vi "configureTiming.vi"(8 "error in (no error)":errorcluster, 9 "Routings":cluster{"Master Clock Route":string[]}, 10 "Timing":T1, 11 "DigitalOutput in":refnum<class "DigitalOutput.lvclass">) -> (0 "error out":errorcluster, 3 "DigitalOutput out":refnum<class "DigitalOutput.lvclass">)   [LabVIEW 2011, in "Hardware.lvlib" / "Channels.lvlib" / "DigitalOutput.lvclass"]
uses:
  DigitalOutput.lvclass
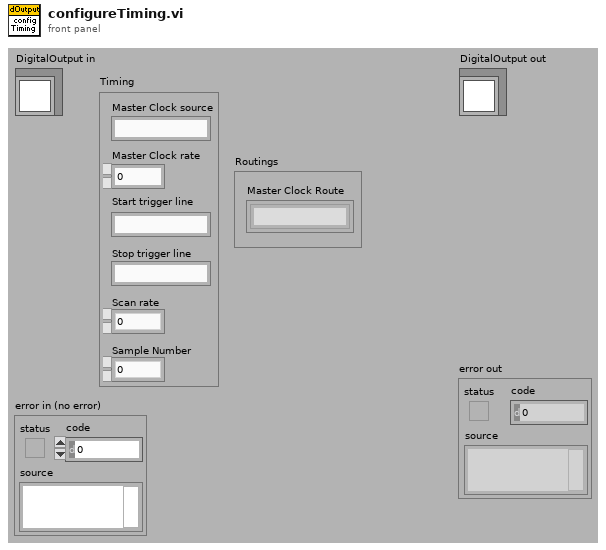
[diagram p1: front panel]
types:
  T1 = cluster{"Master Clock source":string, "Master Clock rate":dbl, "Start trigger line":string, "Scan rate":dbl, "Stop trigger line":string, "Sample Number":dbl}
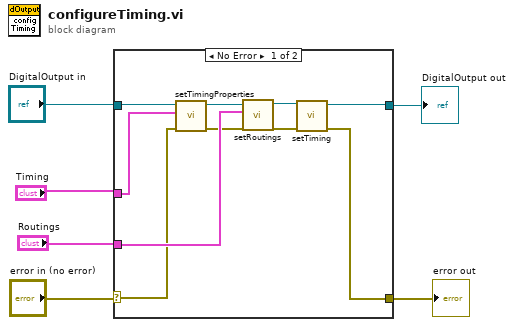
[diagram p0: block diagram]
diagram:
  n1 = case shown="No Error" "error in (no error)" {
    selector: "error in (no error)" -> [w13 w18]
    tunnel: [w7 w18] -> w5
    tunnel: [w8 w17] -> w3
    tunnel: "DigitalOutput in" -> [w12 w17]
    tunnel: "Timing" -> [w11 _]
    tunnel: "Routings" -> [w15 _]
    frame No Error {
      n2 = call-dynamic "setTimingProperties.vi"("error in (no error)"=w13, "Timing"=w11, "DigitalOutput.lvclass in"=w12) -> ("error out"=w14:errorcluster, "DigitalOutput.lvclass out"=w16:refnum<class "DigitalOutput.lvclass">)  [unwired: 7 in]
      n3 = call-dynamic "setRoutings.vi"("error in (no error)"=w14, "Routings"=w15, "DigitalOutput.lvclass in"=w16) -> ("error out"=w10:errorcluster, "DigitalOutput.lvclass out"=w9:refnum<class "DigitalOutput.lvclass">)  [unwired: 7 in]
      n4 = call-dynamic "setTiming.vi"("error in (no error)"=w10, "DigitalOutput in"=w9) -> ("error out"=w7:errorcluster, "DigitalOutput out"=w8:refnum<class "DigitalOutput.lvclass">)  [unwired: 8 in]
    }
    frame Error {
    }
  }
  "error out" <- w5
  "DigitalOutput out" <- w3
